vi "Chamber_and_Multiple_DUTs_Welcome Dialog.vi"() -> ()   [LabVIEW 2015]
doc: "TestStand Chamber and Multiple DUTs example welcome dialog.\n____\nDelacor QMH Thermal Chamber Examples 4.0.0.21\nCopyright (c) 2018, Delacor"
panel:
  in  "Close":bool
  # "Welcome to the Delacor Queued Message Handler TestStand Thermal Chamber Controller Example with multiple DUTs.\n\nThis example executes using the Batch process model file.\n\nThe example contains two DQMH modules\n- Thermal Chamber Controller module (singleton DQMH)\n- Device Under Test module (cloneable DQMH)\n\nTo execute a single instance of the Device Under Test DQMH module run the TestStand Thermal Chamber Controller With DUT.seq example."
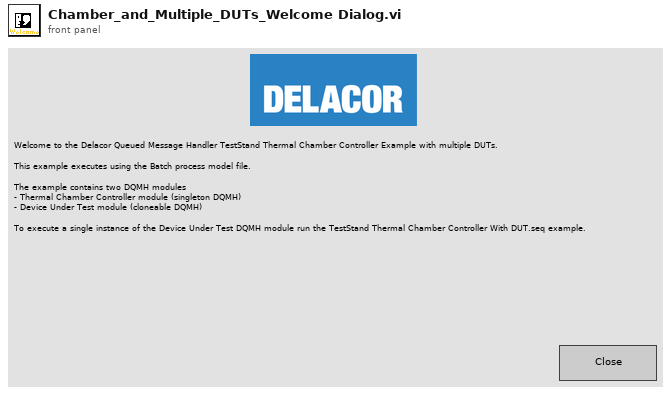
[diagram p1: front panel]
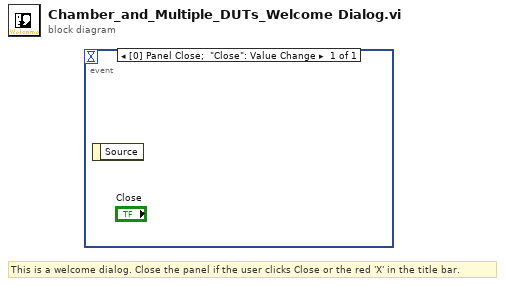
[diagram p0: block diagram]
diagram:
  # "This is a welcome dialog. Close the panel if the user clicks Close or the red 'X' in the title bar."
  n1 = event shown="[0] Panel Close;  \"Close\": Value Change" {
    selector: _ -> [_]
    dyn-events: _ -> [_]
    timeout: _ -> [_]
    event Panel Close; "Close": Value Change {
      n2 = event-data() -> ()  [unwired: 1 in, 1 out]
    }
  }
